vi "test-trapezoid-profile-execute.vi"() -> ()   [LabVIEW 2019]
uses:
  <vilib>/Rock Robotics/WPI/ThirdParty/JAS_Junk/TrajLib/LinearFilter_ResetToValue.vi
  <vilib>/Rock Robotics/WPI/ThirdParty/JAS_Junk/TrajLib/LinearFilter_Calculate.vi
  <vilib>/Rock Robotics/WPI/ThirdParty/JAS_Junk/TrajLib/TrapProfile_Calculate.vi
  <vilib>/Rock Robotics/WPI/ThirdParty/JAS_Junk/TrajLib/TrapProfile_New.vi
  <vilib>/Rock Robotics/WPI/ThirdParty/JAS_Junk/TrajLib/TrapProfile_TotalTime.vi
  <vilib>/Rock Robotics/WPI/ThirdParty/JAS_Junk/TrajLib/TrapProfConstraint_New.vi
  <vilib>/Rock Robotics/WPI/ThirdParty/JAS_Junk/TrajLib/TrapProfState_New.vi
  <vilib>/Rock Robotics/WPI/ThirdParty/JAS_Junk/TrajLib/TrapProfile_Direct.vi
  <vilib>/Rock Robotics/WPI/ThirdParty/JAS_Junk/TrajLib/TrapProfile_ShouldFlipAcceleration.vi
  <vilib>/Rock Robotics/SystemInterfaces/NetworkCommunication/NetComm_UsageReport_report.vi
  <vilib>/Rock Robotics/WPI/ThirdParty/JAS_Junk/TrajLib/LinearFilter_MovingAverage.vi
  <vilib>/Rock Robotics/WPI/ThirdParty/JAS_Junk/TrajLib/LinearFilter_LowPassBW1.vi
  <vilib>/Rock Robotics/WPI/ThirdParty/JAS_Junk/TrajLib/LinearFilter_LowPassBW2.vi
  <vilib>/Rock Robotics/WPI/ThirdParty/JAS_Junk/TrajLib/LinearFilter_HighPassBW1.vi
  <vilib>/Rock Robotics/WPI/ThirdParty/JAS_Junk/TrajLib/LinearFilter_HighPassBW2.vi
  <vilib>/Rock Robotics/WPI/ThirdParty/JAS_Junk/TrajLib/Util_LibraryGlobals.vi
  <vilib>/Rock Robotics/WPI/ThirdParty/JAS_Junk/TrajLib/Trajectory_Library.lvlib
panel:
  out "LibUsage_ProfiledPID":i32 format="%20.0f"
  out "LibUsage_PIDController":i32 format="%20.0f"
  out "LibUsage_Odometry":i32 format="%20.0f"
  out "LibUsage_LinearFIlter":i32 format="%20.0f"
  out "LibUsage_TrapezoidProfile":i32 format="%20.0f"
  out "LibUsage_Kinematics":i32 format="%20.0f"
  out "ActVel":dbl
  out "ActAccel":dbl
  out "ElapsedTIme":dbl format="%20.6f"
  in  "Position\nGoal":dbl=2.0 format="%#_13g"
  out "EstTimeLeft":dbl format="%23.3f"
  out "VelocityDmd":dbl
  out "PositionDmd":dbl
  out "Waveform Chart":T1(graph)
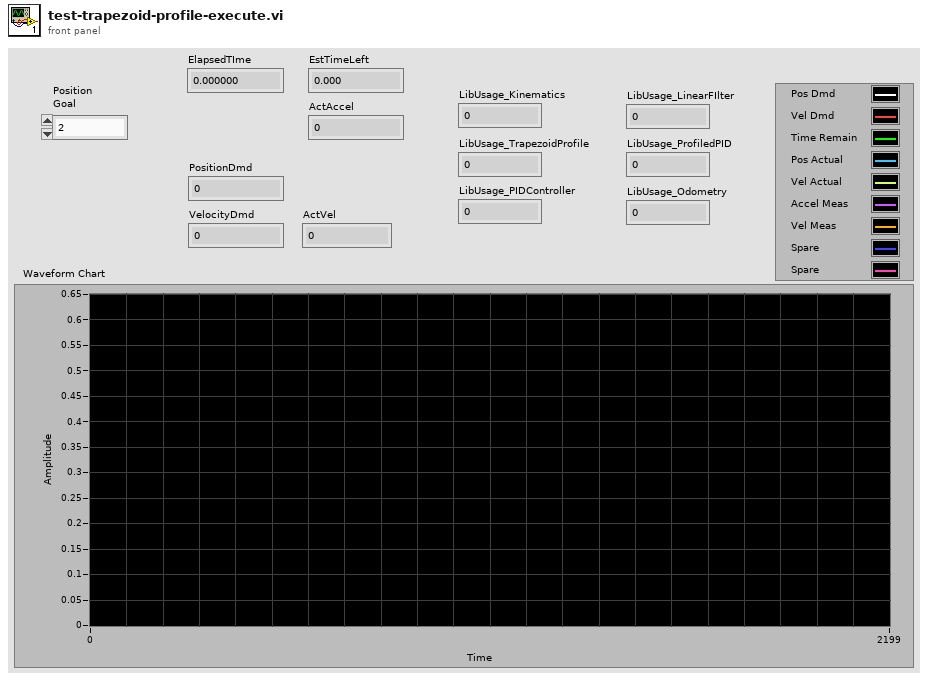
[diagram p1: front panel]
types:
  T1 = cluster{"PositionDmd":dbl, "VelocityDmd":dbl, "EstTimeLeft":dbl, "Output":dbl, "Output":dbl, dbl, dbl, dbl, dbl}
  T2 = enum16{"Moving Average", "Low Pass 1st Order Butterworth", "Low Pass 2nd Order Butterworth", "High Pass 1st Order Butterworth", "High Pass 2nd Order Butterworth"}
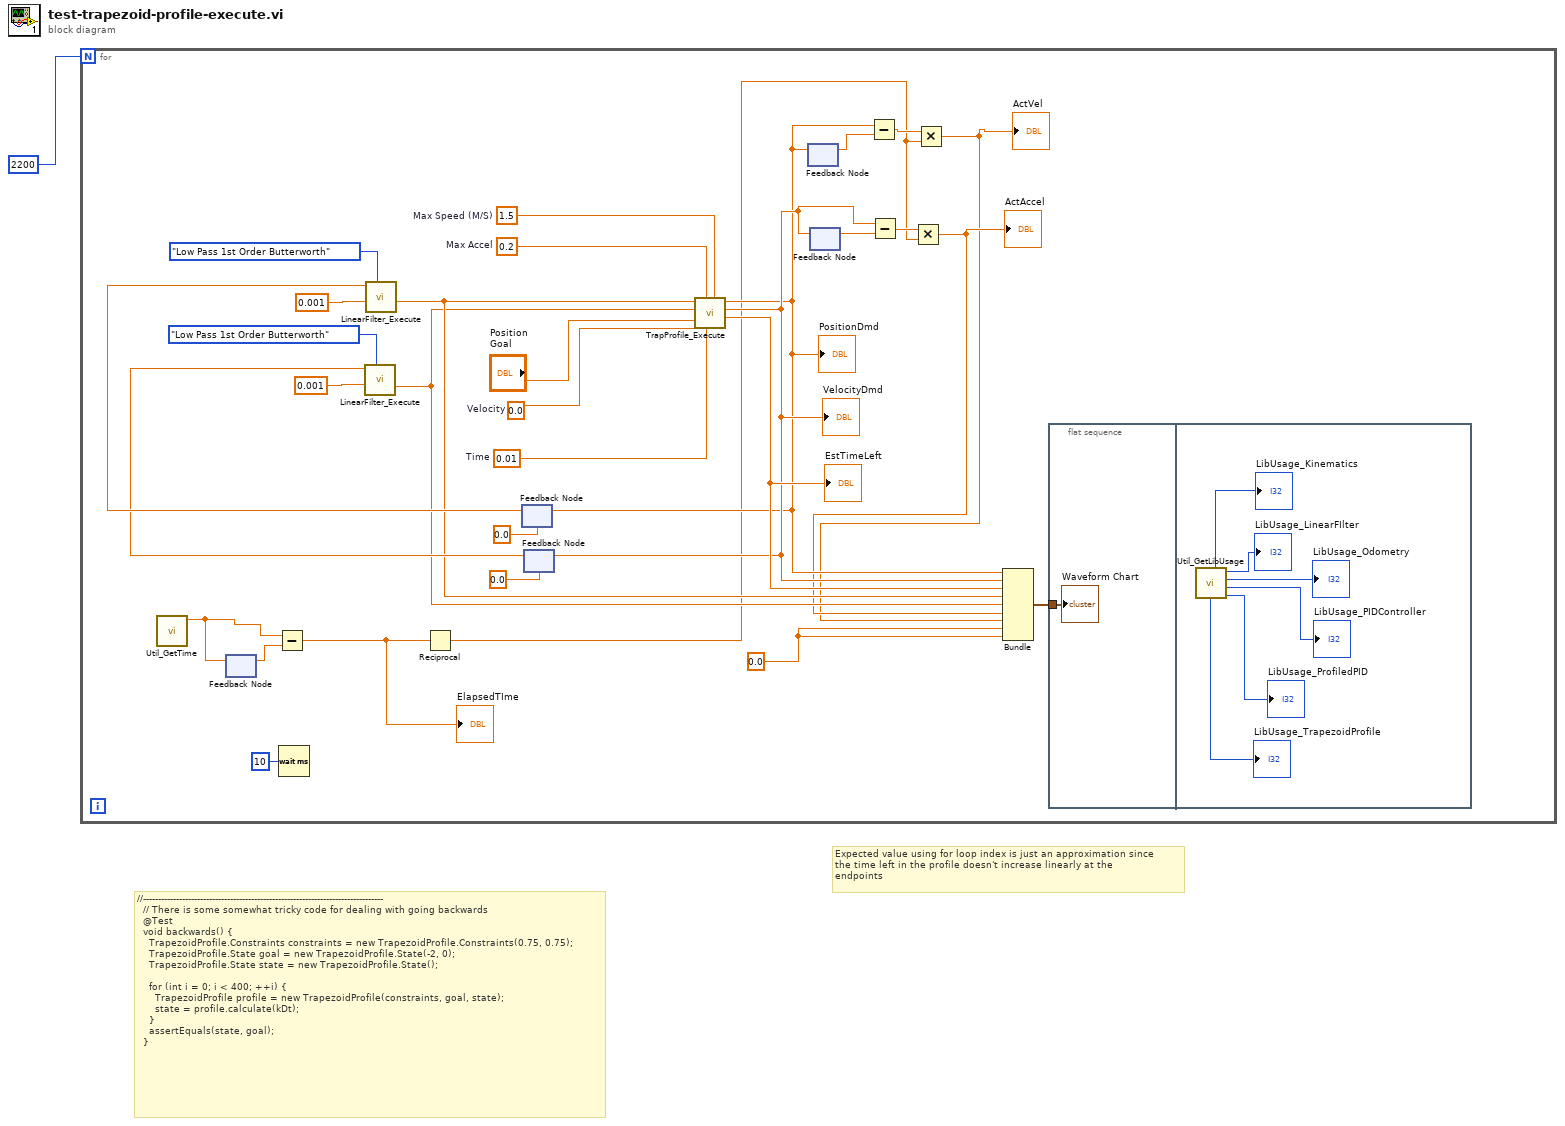
[diagram p0: block diagram]
diagram:
  # "Expected value using for loop index is just an approximation since\nthe time left in the profile doesn't increase linearly at the\nendpoints"
  # "//--------------------------------------------------------------------------------\n  // There is some somewhat tricky code for dealing with going backwards\n  @Test\n  void backwards() {\n    TrapezoidProfile.Constraints constraints = new TrapezoidProfile.Constraints(0.75, 0.75);\n    TrapezoidProfile.State goal = new TrapezoidProfile.State(-2, 0);\n    TrapezoidProfile.State state = new TrapezoidProfile.State();\n\n    for (int i = 0; i < 400; ++i) {\n      TrapezoidProfile profile = new TrapezoidProfile(constraints, goal, state);\n      state = profile.calculate(kDt);\n    }\n    assertEquals(state, goal);\n  }"
  n1 = for {
    N: 2200 -> [_]
    w10 = 0.0
    w28 = 0.0  # Velocity
    w30 = 0.2  # Max Accel
    w31 = 1.5  # Max Speed (M/S)
    w29 = 0.01  # Time
    n2 = call <vilib>:"Util_GetTime.vi"() -> ("FPGA_Time_Seconds"=w14:dbl)  [unwired: 9 in, 2 out]
    n3 = feedback-in #1(w14) -> ()
    n4 = feedback #1() -> (w13:dbl)  [unwired: 1 in]
    n5 = Subtract(x=w14, y=w13) -> (x-y=w7:dbl)
    "ElapsedTIme" <- w7
    n6 = Wait (ms)(milliseconds to wait=u32 10) -> ()  [unwired: 1 out]
    n7 = Reciprocal(x=w7) -> (1/x=w2:dbl)
    n8 = feedback #2(0.0 ("PositionDmd")) -> (w25:dbl)
    n9 = call <vilib>:"LinearFilter_Execute.vi"("Filter Type"=T2."Low Pass 1st Order Butterworth", "TimeConstant"=0.001, "Input"=w25) -> ("Output"=w19:dbl)  [unwired: 7 in, 1 out]
    n10 = feedback #3(0.0 ("VelocityDmd")) -> (w21:dbl)
    n11 = call <vilib>:"LinearFilter_Execute.vi"("Filter Type"=T2."Low Pass 1st Order Butterworth", "TimeConstant"=0.001, "Input"=w21) -> ("Output"=w18:dbl)  [unwired: 7 in, 1 out]
    n12 = call <vilib>:"TrapProfile_Execute.vi"("Max Speed (M/S)"=w31, "TimePeriod"=w29, "Max Accel"=w30, "GoalVelocity"=w28, "GoalPosition"="Position\nGoal", "CurrentVelocity"=w18, "CurrentPosition"=w19) -> ("EstTimeLeft"=w20:dbl, "VelocityDmd"=w11:dbl, "PositionDmd"=w8:dbl)  [unwired: 2 in]
    "PositionDmd" <- w8
    "VelocityDmd" <- w11
    "EstTimeLeft" <- w20
    n13 = feedback-in #2(w8) -> ()
    n14 = feedback-in #3(w11) -> ()
    n15 = feedback #4() -> (w9:dbl)  [unwired: 1 in]
    n16 = feedback-in #4(w8) -> ()
    n17 = feedback #5() -> (w12:dbl)  [unwired: 1 in]
    n18 = feedback-in #5(w11) -> ()
    n19 = Subtract(x=w8, y=w9) -> (x-y=w4:dbl)
    n20 = Subtract(x=w11, y=w12) -> (x-y=w3:dbl)
    n21 = Multiply(x=w3, y=w2) -> (x*y=w6:dbl)
    "ActAccel" <- w6
    n22 = Multiply(x=w4, y=w2) -> (x*y=w5:dbl)
    "ActVel" <- w5
    n23 = Bundle("PositionDmd"=w8, "VelocityDmd"=w11, "EstTimeLeft"=w20, "Output"=w19, "Output"=w18, w6, w5, w10, w10) -> (w17:T1)  [unwired: 1 in]
    n24 = flat-sequence {
      tunnel: w17 -> [w33]
      frame #0 {
        "Waveform Chart" <- w33
      }
      frame #1 {
        n25 = call <vilib>:"Util_GetLibUsage.vi"() -> ("LibUsage_ProfiledPID"=→"LibUsage_ProfiledPID":i32, "LibUsage_PIDController"=→"LibUsage_PIDController":i32, "LibUsage_Odometry"=→"LibUsage_Odometry":i32, "LibUsage_LinearFIlter"=→"LibUsage_LinearFIlter":i32, "LibUsage_TrapezoidProfile"=→"LibUsage_TrapezoidProfile":i32, "LibUsage_Kinematics"=→"LibUsage_Kinematics":i32)  [unwired: 6 in]
      }
    }
  }
